vi "get_PV.vi"(0 "HGF_NetworkData":refnum<class "HGF_NetworkVisitor.lvclass">, 5 "error in (no error)":errorcluster) -> (14 "dup HGF_NetworkData":refnum<class "HGF_NetworkVisitor.lvclass">, 16 "HGV_PVBase":refnum<class "HGF_PVBase.lvclass">, 19 "error out":errorcluster)   [LabVIEW 2014, in "HGF_BaseClasses.lvlib" / "HGF_NetworkVisitor.lvclass"]
uses:
  HGF_NetworkVisitor.lvclass
  HGF_PVBase/HGF_PVBase.lvclass
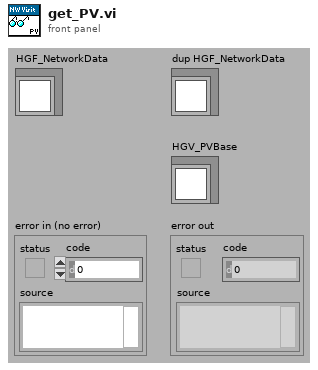
[diagram p1: front panel]
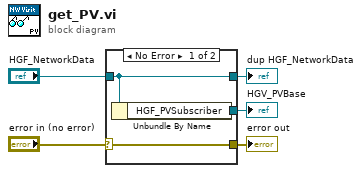
[diagram p0: block diagram]
diagram:
  n1 = case shown="No Error" "error in (no error)" {
    selector: "error in (no error)" -> [w8 w9]
    tunnel: [w8 w9] -> w4
    tunnel: [w7 w10] -> w2
    tunnel: "HGF_NetworkData" -> [w7 w10]
    tunnel: [w6 _] -> w1
    frame No Error {
      n2 = Unbundle By Name(w7) -> ("HGF_PVSubscriber"=w6:refnum<class "HGF_PVSubscriber.lvclass">)
    }
    frame Error {
    }
  }
  "error out" <- w4
  "dup HGF_NetworkData" <- w2
  "HGV_PVBase" <- w1
